vi "Read Value Type.vi"(8 "error in (no error)":errorcluster, 11 "DriverSetting in":refnum<class "DriverSetting.lvclass">) -> (0 "error out":errorcluster, 2 "Value Type":string, 3 "DriverSetting out":refnum<class "DriverSetting.lvclass">)   [LabVIEW 2023, in "HAF.lvlib" / "DriverSetting.lvclass"]
doc: "Returns the data type of the Driver Settings Value. Must be in the list of Valid Data Types."
uses:
  DriverSetting.lvclass
  DriverSetting.lvclass/DriverSetting.ctl
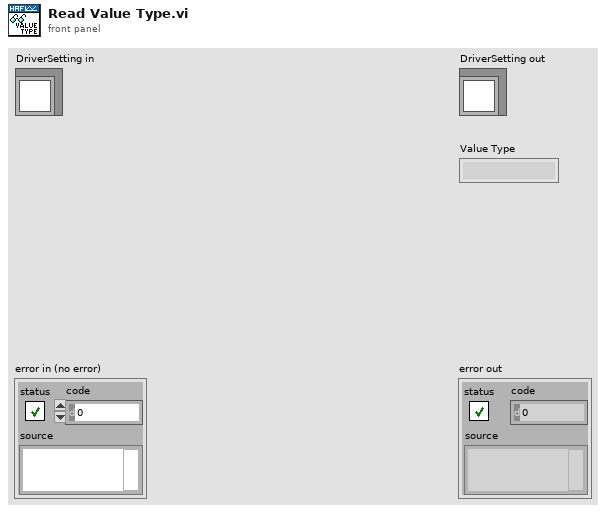
[diagram p1: front panel]
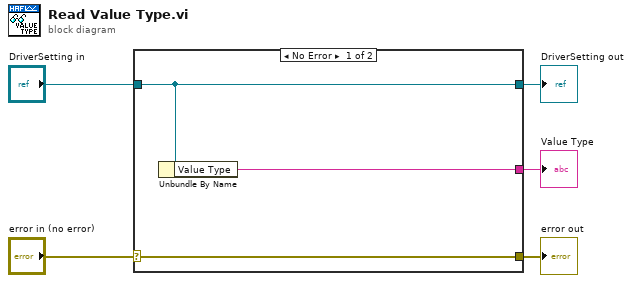
[diagram p0: block diagram]
diagram:
  n1 = case shown="No Error" "error in (no error)" {
    selector: "error in (no error)" -> [w8 w9]
    tunnel: [w8 w9] -> w4
    tunnel: [w7 w10] -> w2
    tunnel: "DriverSetting in" -> [w7 w10]
    tunnel: [w6 _] -> w1
    frame No Error {
      n2 = Unbundle By Name(w7) -> ("Value Type"=w6:string)
    }
    frame Error {
    }
  }
  "error out" <- w4
  "DriverSetting out" <- w2
  "Value Type" <- w1
